vi "Close.vi"(8 "error in":errorcluster, 11 "Cell in":refnum<class "Cell.lvclass">) -> (0 "error out":errorcluster, 3 "Cell out":refnum<class "Cell.lvclass">)   [LabVIEW 2023, in "SourceGrid.lvlib" / "Cell.lvclass"]
uses:
  Cell.lvclass
  Cell.lvclass/Cell.ctl
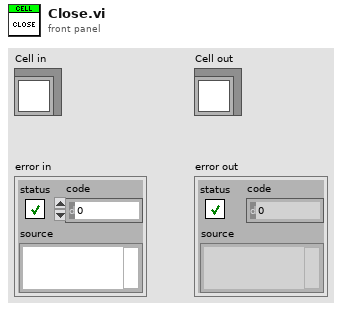
[diagram p1: front panel]
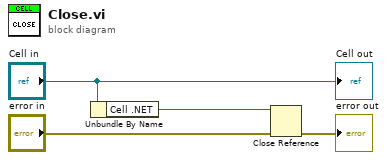
[diagram p0: block diagram]
diagram:
  n1 = Unbundle By Name("Cell in") -> ("Cell .NET"=w3:refnum<k24>)
  n2 = Close Reference(reference=w3, error in (no error)="error in") -> (error out=→"error out":errorcluster)
  "Cell out" <- "Cell in"
